vi "Example_plot_isoteric_chart.vi"(7 "W-Array in kg/kg (Input)":dbl[](array[numeric])=[0.01, 0.025, 0.1, 0.2, 0.3, 0.4, 0.5], 9 "T_max in K (Input)":dbl=647.0, 10 "T_min in K (Input)":dbl=283.15, 11 "WorkingPair (Input)":T1={"no_iso"=1, "no_p_sat"=1, "path_db"="D:\\Driesel\\SorpLibLocal\\labview_wrapper\\data\\json\\sorpproplib.json", "wp_as"="silica gel pellet", "wp_st"="123", "wp_iso"="DubininArctan1", "wp_rf"="Water", "rf_rhol"="SaturatedLiquidDensity_EoS1", "no_rhol"=1, "rf_psat"="VaporPressure_EoS1"}) -> ()   [LabVIEW 2017]
panel:
  out "Isosteres":cluster{dbl[], dbl[]}[](graph)=[{array[365 elements], array[365 elements]}, {array[365 elements], array[365 elements]}, {array[365 elements], array[365 elements]}, {array[365 elements], array[365 elements]}, {array[359 elements], array[359 elements]}, {array[289 elements], array[289 elements]}, {[-0.003531696980399082, -0.0035192679922576107, -0.0035069261792039282, -0.003494670627293378, -0.0034825004353125546, -0.00347041471455839, -0.003458412588621823, -0.0034464931931759437, -0.0034346556757685045, -0.0034228991956186893, -0.003411222923418046, -0.0033996260411354754, -0.0033881077418261903, -0.0033766672294445383, -0.0033653037186606094, -0.0033540164346805303, -0.003342804613070366, -0.003331667499583542, -0.003320604349991699, -0.0033096144299189145, -0.003298697014679202, -0.003287851389117212, -0.003277076847452073, -0.003266372693124286, -0.003255738238645613, -0.0032451728054518907, -0.0032346757237586934, -0.003224246332419797, -0.003213883978788366, -0.0032035880185808108, -0.003193357815743254, -0.0031831927423205475, -0.0031730921783277807, -0.003163055511624229, -0.0031530821377896896, -0.0031431714600031434, -0.0031333228889237038, -0.003123535842573794, -0.0031138097462245057, -0.003104144032283098, -0.0030945381401825778, -0.0030849915162733305, -0.0030755036137167465, -0.0030660738923808067, -0.0030567018187375823, -0.0030473868657626088, -0.0030381285128360932, -0.003028926245645919, -0.0030197795560924054, -0.0030106879421947915, -0.0030016509079994, -0.002992667963489451, -0.002983738624496494, -0.002974862412613417, -0.002966038855109002, -0.0029572674848440043, -0.0029485478401887074, -0.0029398794649419377, -0.0029312619082515023, -0.0029226947245360223, -0.002914177473408131, -0.002905709719599012, -0.0028972910328842532, -0.0028889209880109783, -0.0028805991646262425, -0.002872325147206664, -0.0028640985249892598, -0.00285591889190347, -0.002847785846504343, -0.002839698991906858, -0.002831657935721365, -0.002823662289990117, -0.002815711671124877, -0.002807805699845571, -0.0027999440011199778, -0.002792126204104426, -0.00278435194208548, -0.0027766208524226017, -0.0027689325764917627, -0.0027612867596299878, -0.002753683051080821, -0.002746121103940684, -0.002738600575106121, -0.0027311211252219036, -0.0027236824186299877, -0.0027162841233192994, -0.0027089259108763375, -0.00270160745643658, -0.00269432843863667, -0.002687088539567379, -0.0026798874447273215, -0.0026727248429774158, -0.0026656004264960682, -0.0026585138907350794], [995.6868807653667, 1065.5938991149683, 1139.8574391068994, 1218.7117814882488, 1302.401645095998, 1391.1825454296695, 1485.3211613320625, 1585.0957098471665, 1690.7963293242678, 1802.7254708382966, 1921.1982979968375, 2046.5430952054487, 2179.1016844642027, 2319.229850770136, 2467.297776201945, 2623.690482765518, 2788.808284081765, 2963.067246000752, 3146.899656229439, 3340.7545030642627, 3545.0979633235356, 3760.4138995790445, 3987.2043667916496, 4225.990128460064, 4477.311182398888, 4741.727296267391, 5019.818552977553, 5312.185906117583, 5619.451745534454, 5942.260473227631, 6281.279089715428, 6637.197791044433, 7010.730576623637, 7402.615868075008, 7813.6171393044415, 8244.523558008743, 8696.150638848858, 9169.34090853134, 9664.964583056706, 10183.920257407988, 10727.135607969129, 11295.568107981539, 11890.205756363213, 12512.067820236784, 13162.205591531703, 13841.703158047952, 14551.678189391017, 15293.282738212663, 16067.704057216224, 16876.165432412705, 17719.927033141066, 18600.286779396734, 19518.581227041646, 20476.186471504287, 21474.519070609156, 22515.036987215448, 23599.240552378036, 24728.673449789396, 25904.923722296717, 27129.624801339716, 28404.456560195467, 29731.146391970313, 31111.470313326685, 32547.25409499115, 34040.37442014383, 35592.76007185284, 37206.393150778495, 38883.310324442566, 40625.60410942416, 42435.42418792465, 44314.97876021472, 46266.53593457144, 48292.42515638591, 50395.03867823235, 52576.83307276827, 54840.33079046082, 57188.121764219315, 59622.8650631532, 62147.29059777922, 64764.20087914201, 67476.47283444299, 70287.0596819237, 73198.99286789467, 76215.38406897619, 79339.42726277668, 82574.40087043002, 85923.66997459781, 89390.68861675632, 92979.00217780344, 96692.2498462531, 100534.16717853813, 104508.58875619763, 108619.45094501246, 112870.79476144738]}, {[], []}]
  # "Path to database"
  # "Name of sorbent"
  # "Name of sub-type of sorbent"
  # "Name of refrigerant"
  # "Name of isotherm"
  # "ID of isotherm"
  # "Name of calculation approach for vapor pressure"
  # "ID of vapor pressure equation"
  # "Name of calculation approach for liquid density"
  # "ID of liquid density equation"
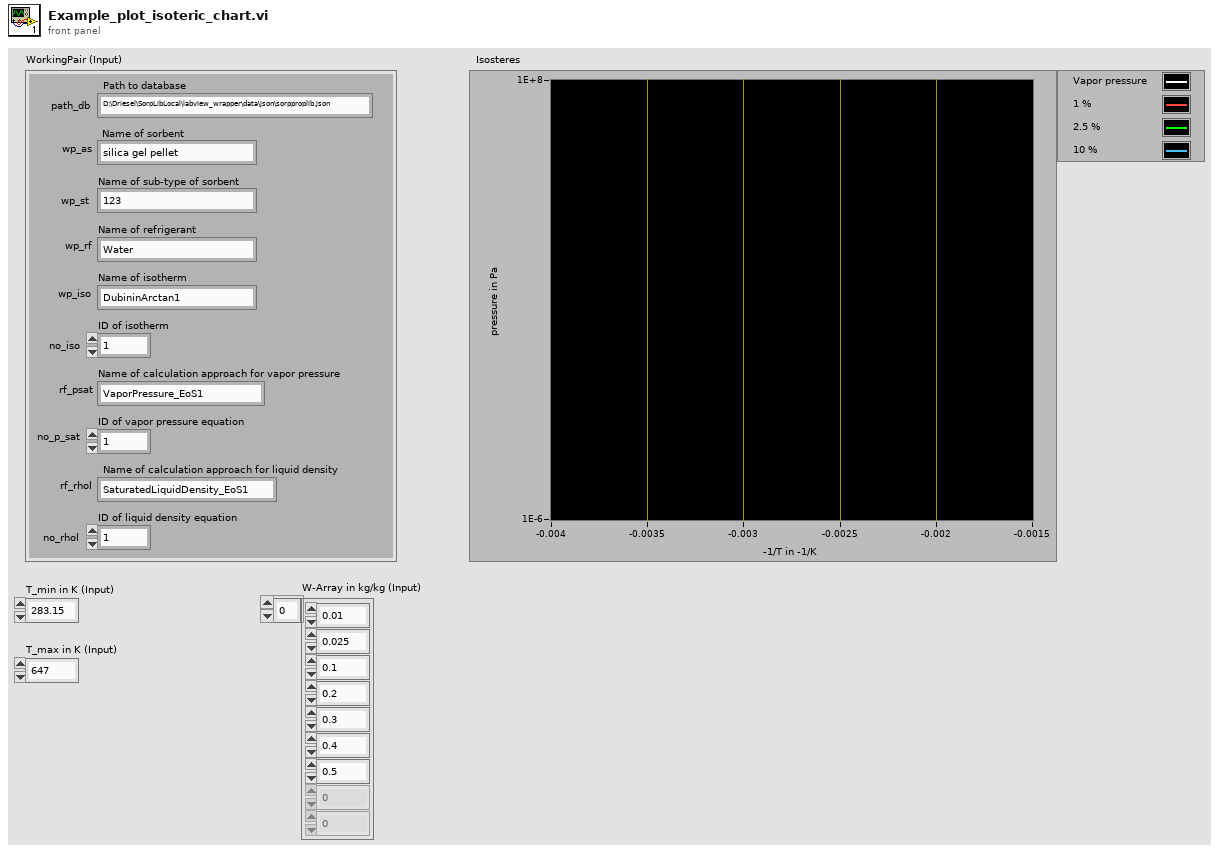
[diagram p1: front panel]
types:
  T1 = cluster{"no_iso":i32, "no_p_sat":i32, "path_db":string, "wp_as":string, "wp_st":string, "wp_iso":string, "wp_rf":string, "rf_rhol":string, "no_rhol":i32, "rf_psat":string}
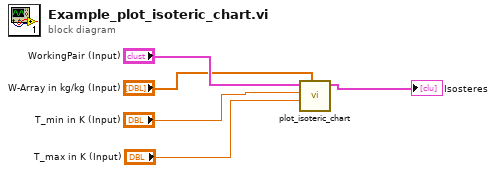
[diagram p0: block diagram]
diagram:
  n1 = call "plot_isoteric_chart.vi"("W-Array in kg/kg (Input)"="W-Array in kg/kg (Input)", "T_max in K (Input)"="T_max in K (Input)", "T_min in K (Input)"="T_min in K (Input)", "WorkingPair (Input)"="WorkingPair (Input)") -> ("Isosteres"=→"Isosteres":cluster{dbl[], dbl[]}[])  [unwired: 6 in, 1 out]
